vi "AFG3031.vi"() -> (0 "Reading":dbl)   [LabVIEW 2010]
uses:
  <vilib>/Instr/_visa.llb/VISA Configure Serial Port (Instr).vi
panel:
  out "read buffer":string
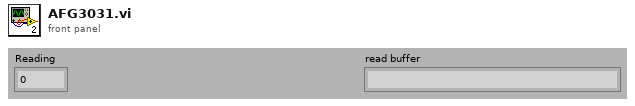
[diagram p1: front panel]
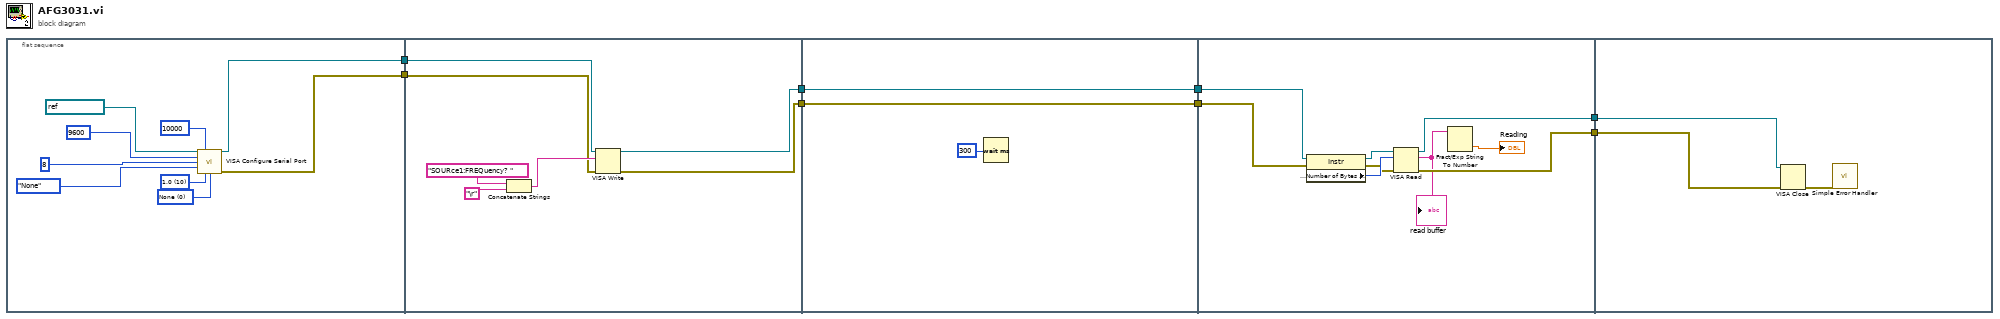
[diagram p0: block diagram]
diagram:
  n1 = flat-sequence {
    tunnel: [w10] -> w8
    tunnel: [w9] -> w7
    tunnel: w8 -> [w21]
    tunnel: w7 -> [w20]
    tunnel: [w19] -> w6
    tunnel: [w18] -> w5
    tunnel: w6 -> [w26]
    tunnel: [w26] -> w4
    tunnel: w5 -> [w25]
    tunnel: [w25] -> w3
    tunnel: w4 -> [w33]
    tunnel: w3 -> [w32]
    tunnel: [w31] -> w2
    tunnel: [w30] -> w1
    tunnel: w2 -> [w38]
    tunnel: w1 -> [w37]
    frame #0 {
      w12 = u16 0 items=["None", "XON/XOFF", "RTS/CTS", "XON/XOFF & RTS/CTS", "DTR/DSR", "XON/XOFF & DTR/DSR"] ("flow control (0:none)")
      w13 = u16 10 items=["1.0"=10, "1.5"=15, "2.0"=20] ("stop bits (10: 1 bit)")
      n2 = call-poly "VISA Configure Serial Port"("VISA resource name"=refnum<visa-resource-name> "AFG3031", "timeout (10sec)"=u32 10000, "baud rate (9600)"=u32 9600, "data bits (8)"=u16 8, "parity (0:none)"=enum16{"None", "Odd", "Even", "Mark", "Space"}."None", "stop bits (10: 1 bit)"=w13, "flow control (0:none)"=w12) -> ("VISA resource name out"=w10:refnum<visa-resource-name>, "error out"=w9:errorcluster)  [unwired: 2 in, 5 out]
    }
    frame #1 {
      n3 = Concatenate Strings("SOURce1:FREQuency? ", "\r") -> (w22:string)
      n4 = VISA Write(VISA resource name=w21, write buffer=w22, error in (no error)=w20) -> (VISA resource name out=w19:refnum<visa-resource-name>, error out=w18:errorcluster)  [unwired: 1 out]
    }
    frame #2 {
      n5 = Wait (ms)(milliseconds to wait=u32 300) -> ()  [unwired: 1 out]
    }
    frame #3 {
      n6 = property class="Instr"(reference=w33, error in=w32) -> (reference out=w36:refnum<visa-resource-name>, error out=w34:errorcluster, "Serial Settings:Number of Bytes at Serial Port"=w35:u32)
      n7 = VISA Read(VISA resource name=w36, byte count=w35, error in (no error)=w34) -> (VISA resource name out=w31:refnum<visa-resource-name>, read buffer=w29:string, error out=w30:errorcluster)  [unwired: 1 out]
      "read buffer" <- w29
      n8 = Fract/Exp String To Number(string=w29) -> (number=→"Reading":dbl)  [unwired: 3 in, 1 out]
    }
    frame #4 {
      n9 = VISA Close(VISA resource name=w38, error in (no error)=w37) -> (error out=w39:errorcluster)
      n10 = call <vilib>:"Simple Error Handler.vi"("error in (no error)"=w39) -> ()  [unwired: 1 in, 8 out]
    }
  }
